vi "音频操作.vi"(7 "WindowsMediaPlayer":refnum<k7>(container), 8 "错误输入":errorcluster caption="错误输出", 9 "索引":i32, 11 "选项":enum16{"初始化", "播放声音", "获取寄存器", "关闭播放器"}(ring)) -> (0 "error out":errorcluster, 3 "播放完成":bool)   [LabVIEW 2017]
panel:
  out "status":string
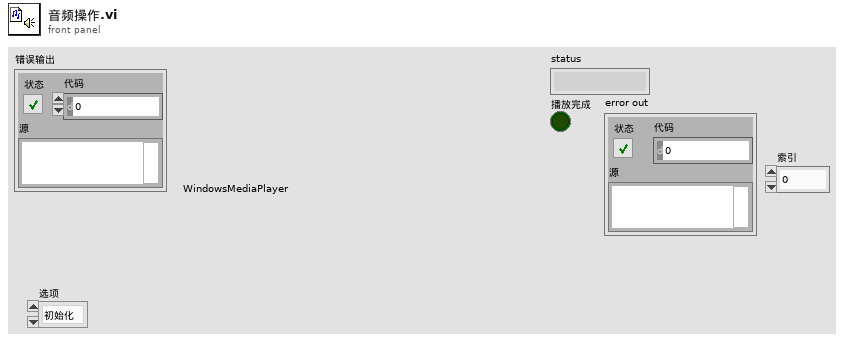
[diagram p1: front panel]
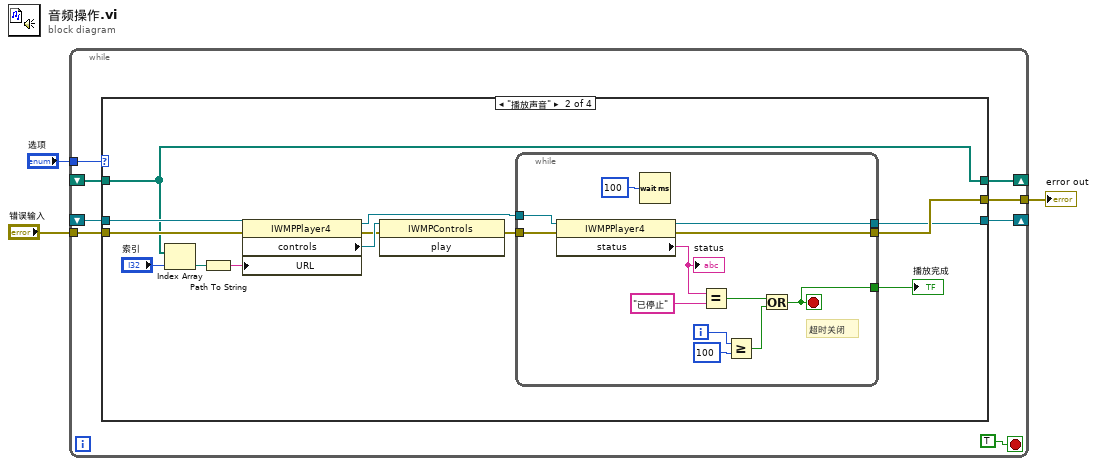
[diagram p0: block diagram]
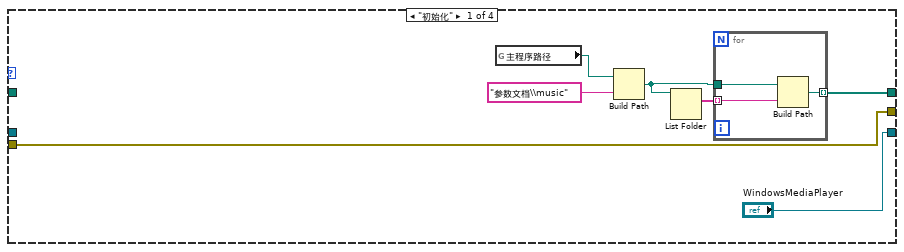
[diagram p2: hidden frame]
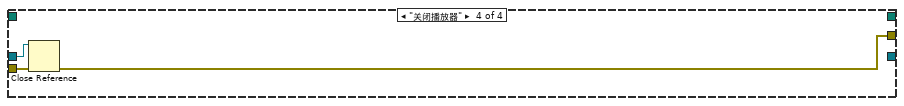
[diagram p4: hidden frame]
diagram:
  n1 = while {
    shift-right: [w6] -> _
    shift-left: _ -> [w10]
    tunnel: "选项" -> [w9]
    tunnel: "错误输入" -> [w8]
    tunnel: [w7] -> w1
    shift-right: [w5] -> _
    shift-left: _ -> [w4]
    stop <- TRUE stop-if-true
    n2 = case shown="\"播放声音\"" w9 {
      tunnel: w10 -> [_ w26 w49 w52]
      tunnel: w8 -> [w13 w25 w47 w51]
      tunnel: [w13 w24 w47 w50] -> w7
      tunnel: ["WindowsMediaPlayer" w23 w49 _] -> w6
      tunnel: [w12 w22 w48 _] -> w5
      tunnel: w4 -> [_ w22 w48 _]
      frame "初始化" {
        n3 = global read "全局 1.vi" "主程序路径"() -> (w18:path)
        n4 = Build Path(base path=w18, name or relative path="参数文档\\music" ("名称或相对路径")) -> (appended path=w15:path)
        n5 = List Folder(path=w15) -> (filenames=w16:string[])  [unwired: 3 in, 3 out]
        n6 = for {
          tunnel: w16 -> [w20] mode=indexing
          tunnel: w15 -> [w21]
          tunnel: [w19] -> w12 mode=indexing
          n7 = Build Path(base path=w21, name or relative path=w20) -> (appended path=w19:path)
        }
      }
      frame "播放声音" {
        n8 = Index Array(array=w22, index="索引") -> (element=w28:path)
        n9 = Path To String(path=w28) -> (string=w31:string)
        n10 = property class="IWMPPlayer4"(reference=w26, error in=w25, "URL"=w31) -> (reference out=w33:refnum<k7>, error out=w32:errorcluster, "controls"=w34:refnum<k7>)
        n11 = invoke class="IWMPControls" method="play"(reference=w34, error in=w32) -> (error out=w30:errorcluster)  [unwired: 1 in, 2 out]
        n12 = while {
          tunnel: w30 -> [w43]
          tunnel: w33 -> [w46]
          tunnel: [w35] -> w27
          tunnel: [w40] -> w24
          tunnel: [w39] -> w23
          i -> [w36]
          stop <- w35 stop-if-true
          # "超时关闭"
          n13 = property class="IWMPPlayer4"(reference=w46, error in=w43) -> (reference out=w39:refnum<k7>, error out=w40:errorcluster, "status"=w45:string)
          "status" <- w45
          n14 = Wait (ms)(milliseconds to wait=u32 100 ("等待时间（毫秒）")) -> ()  [unwired: 1 out]
          n15 = Equal?(x=w45, y="已停止" ("status")) -> (x = y?=w41:bool)
          n16 = Greater Or Equal?(x=w36, y=u32 100) -> (x >= y?=w37:bool)
          n17 = Or(x=w41, y=w37) -> (x .or. y?=w35:bool)
        }
        "播放完成" <- w27
      }
      frame "获取寄存器" {
      }
      frame "关闭播放器" {
        n18 = Close Reference(reference=w52, error in (no error)=w51) -> (error out=w50:errorcluster)
      }
    }
  }
  "error out" <- w1
